vi "Attack.vi"(8 "View":i32[](array[numeric]), 9 "Team Index":i32, 11 "ChargeDirection":T1) -> (0 "Enemy":i32, 1 "Direction":i32, 2 "Action":T2, 4 "Enemy Found?":bool, 6 "Enemy Direction":i32)   [LabVIEW 2020, in "Atom.lvclass"]
uses:
  Atom.lvclass
  Type Defs/Action Enum.ctl
  Type Defs/Direction Enum.ctl
  Type Defs/SB Type Defs.lvlib
  Common/Common.lvlib
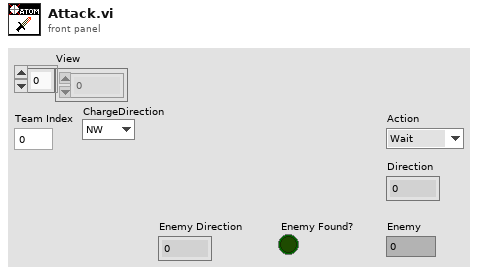
[diagram p1: front panel]
types:
  T1 = typedef "SB Type Defs.lvlib/Direction Enum.ctl" = enum16{"NW", "N", "NE", "E", "SE", "S", "SW", "W"}
  T2 = typedef "SB Type Defs.lvlib/Action Enum.ctl" = enum16{"Wait", "Move", "Attack", "Replicate"}
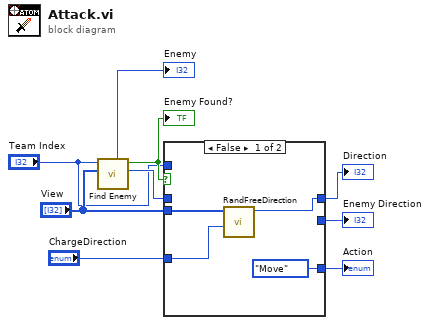
[diagram p0: block diagram]
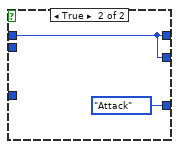
[diagram p2: hidden frame]
diagram:
  n1 = call "Find Enemy.vi"("View"="View", "Team Index"="Team Index") -> ("Direction"=w6:T1, "Found Enemy?"=w5:bool, "Enemy"=→"Enemy":i32)  [unwired: 7 in]
  "Enemy Found?" <- w5
  n2 = case shown="False" w5 {
    tunnel: [Action_Enum."Move" ("Action") Action_Enum."Attack" ("Action")] -> w8
    tunnel: [w11 w14] -> w9
    tunnel: [_ w14] -> w7
    tunnel: w6 -> [_ w14]
    tunnel: "ChargeDirection" -> [w12 _]
    tunnel: "View" -> [w13 _]
    tunnel: "Team Index" -> [_ _]
    frame False {
      n3 = call "RandFreeDirection.vi"("Intended Dir"=w12, "View"=w13) -> ("Direction"=w11:T1)  [unwired: 8 in, 1 out]
    }
    frame True {
    }
  }
  "Action" <- w8
  "Direction" <- w9
  "Enemy Direction" <- w7
